vi "PicoScope4000aStop.vi"(8 "error in (no error)":errorcluster, 11 "handle in":i16=16384) -> (0 "error out":errorcluster, 3 "handle out":i16)   [LabVIEW 2010]
doc: "This stops the device capturing data and should be called before retrieving data from the device."
uses:
  ps4000a.dll
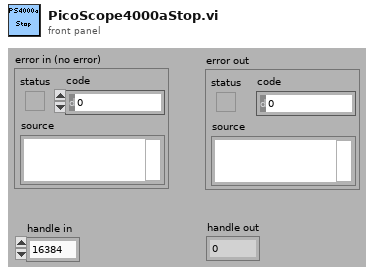
[diagram p1: front panel]
types:
  T1 = cluster{"status":bool, "code":u32, "source":string}
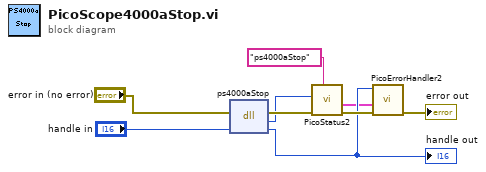
[diagram p0: block diagram]
diagram:
  n1 = dll-call lib="ps4000a.dll" fn="ps4000aStop"(error in="error in (no error)", "handle"="handle in") -> (error out=w9:errorcluster, "PICO_STATUS"=w8:u32, "handle"=w2:i16)  [unwired: 2 in, 1 out]
  "handle out" <- w2
  n2 = call "PicoStatus2.vi"("PICO source"="ps4000aStop" ("source"), "Error in"=w9, "PICO STATUS"=w8) -> ("error out"=w7:errorcluster, "PICO_STATUS out"=w1:T1)  [unwired: 5 in]
  n3 = call "PicoErrorHandler2.vi"("error in (no error)"=w7, "PICO_STATUS in"=w1, "handle In"=w2) -> ("error out"=→"error out":errorcluster)  [unwired: 8 in]
